vi "Introspection Core.vi"(8 "error in (no error)":errorcluster, 11 "CS++StartActor in":refnum<class "CS++StartActor.lvclass">) -> (0 "error out":errorcluster, 2 "CS++Messages":refnum<class "Message.lvclass">[](array[class]), 3 "CS++StartActor out":refnum<class "CS++StartActor.lvclass">)   [LabVIEW 2014, in "CS++StartActor.lvlib" / "CS++StartActor.lvclass"]
doc: "This vi delivers a list with all messages this actor reacts to. \n\nNote that all inherited classes have to overwrite it."
uses:
  CS++StartActor.lvclass
  CS++BaseActor/CS++BaseActor.lvclass
  CS++StartActor Messages/Launch Actors Msg/Launch Actors Msg.lvclass
  CS++StartActor Messages/Launch Start Actors Msg/Launch Start Actors Msg.lvclass
  <vilib>/ActorFramework/Message/Message.lvclass
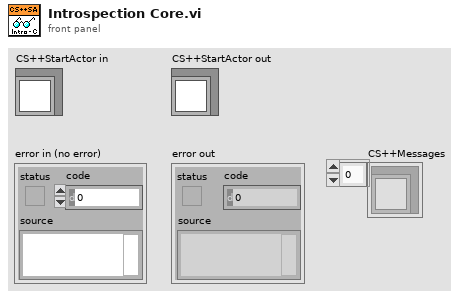
[diagram p1: front panel]
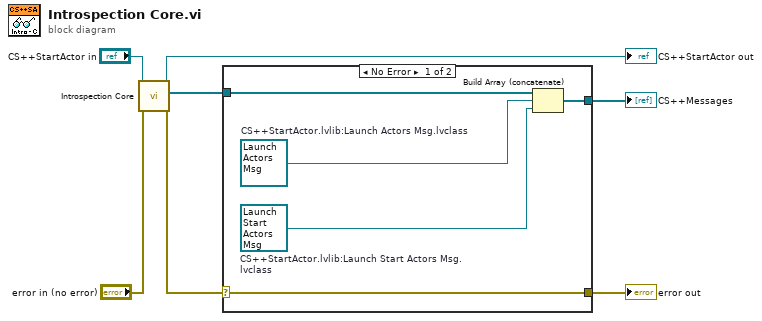
[diagram p0: block diagram]
diagram:
  n1 = call-parent "Introspection Core.vi"("error in (no error)"="error in (no error)", "CS++BaseActor in"="CS++StartActor in") -> ("error out"=w2:errorcluster, "CS++Messages"=w4:refnum<class "Message.lvclass">[], "CS++BaseActor out"=→"CS++StartActor out":refnum<class "CS++StartActor.lvclass">)  [unwired: 7 in]
  n2 = case shown="No Error" w2 {
    selector: w2 -> [w12 w13]
    tunnel: [w12 w13] -> w1
    tunnel: w4 -> [w11 _]
    tunnel: [w8 _] -> w3
    frame No Error {
      w9 = refnum<class "Launch Start Actors Msg.lvclass"> refnum  # CS++StartActor.lvlib:Launch Start Actors Msg.lvclass
      w10 = refnum<class "Launch Actors Msg.lvclass"> refnum  # CS++StartActor.lvlib:Launch Actors Msg.lvclass
      n3 = Build Array (concatenate)(w11, w10, w9) -> (w8:refnum<class "Message.lvclass">[])
    }
    frame Error {
    }
  }
  "error out" <- w1
  "CS++Messages" <- w3
